vi "FinBuild2.vi"   [LabVIEW 2015]
uses:
  <vilib>/NXT/Block Support/NXT_InputPort.ctl
  <vilib>/NXT/Block Support/NXT_OutputPort.ctl
  <vilib>/NXT/Dual Mode Library/Sensors/Light_On.vi
  <vilib>/NXT/Dual Mode Library/Sensors/Sonar_cm.vi
  <vilib>/NXT/NXTIO Xnodes/NXTIONodeSubVIs/NXTMoveMotors.vi
  <vilib>/NXT/Dual Mode Library/Waits/Wait_Num(msec).vi
  <vilib>/NXT/Subs/LVHSConnector.ctl
  <vilib>/NXT/NXTIO Xnodes/AddressXNode/NXTIOAddress.xnode
  <vilib>/NXT/NXTIO Xnodes/NXTIOXNode/NXTIO.xnode
  <vilib>/NXT/LegoClasses/BrickReference/BrickReference.lvclass
types:
  T1 = typedef "NXT_OutputPort.ctl" = u8
  T2 = typedef "NXT_InputPort.ctl" = u32
  T3 = typedef "LVHSConnector.ctl" = refnum<class "BrickReference.lvclass">
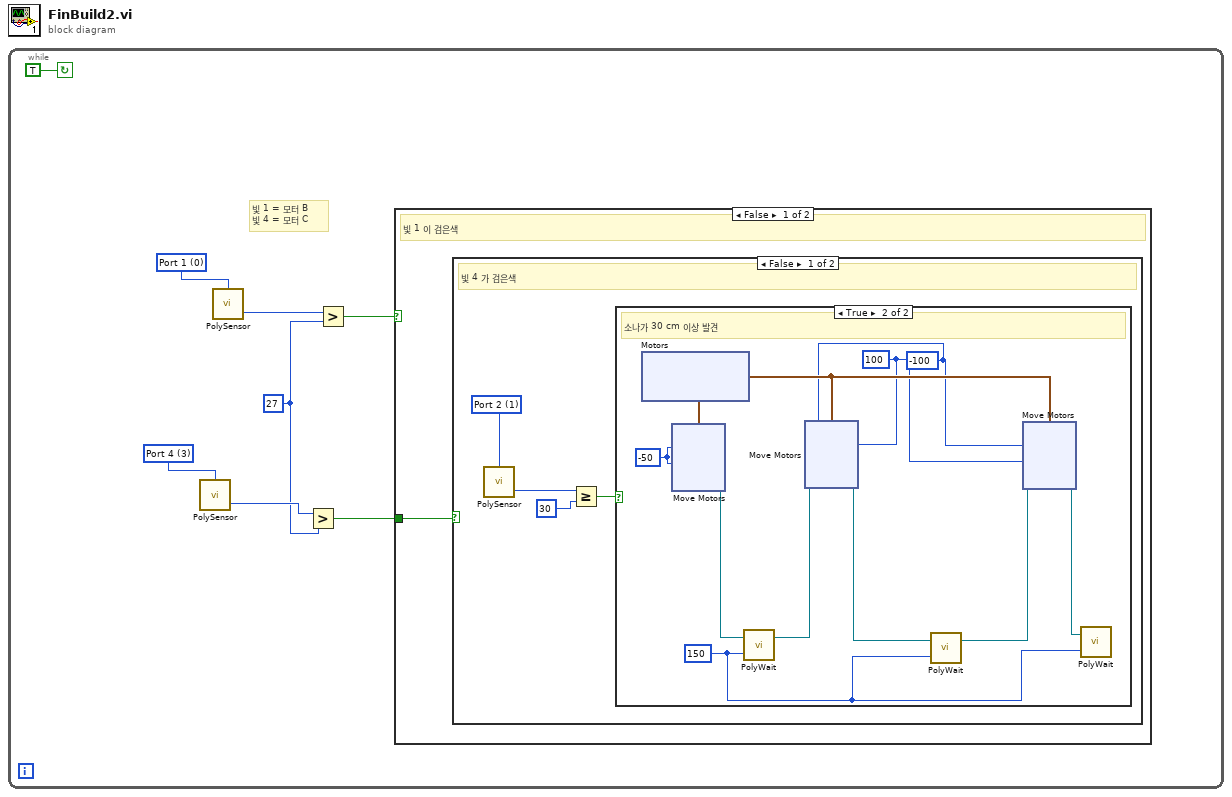
[diagram p0: block diagram]
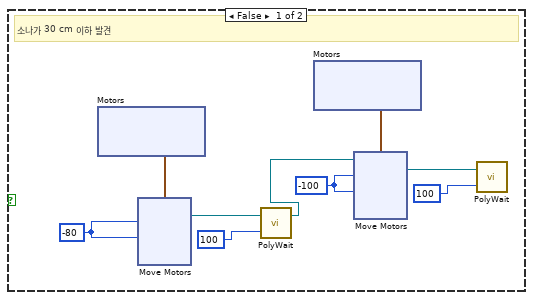
[diagram p2: hidden frame]
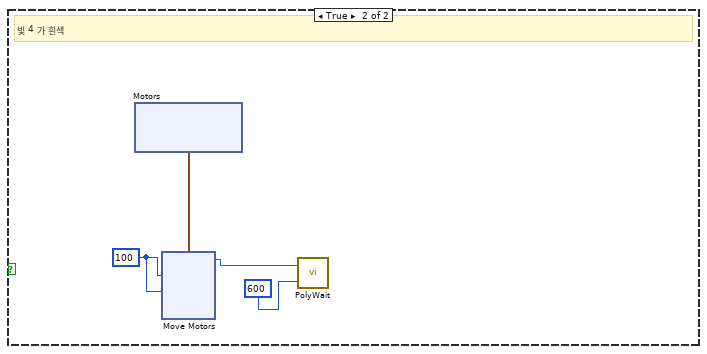
[diagram p3: hidden frame]
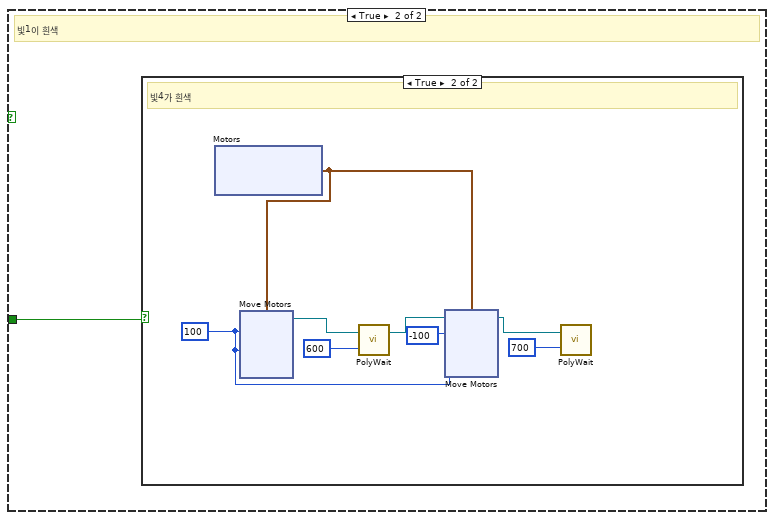
[diagram p4: hidden frame]
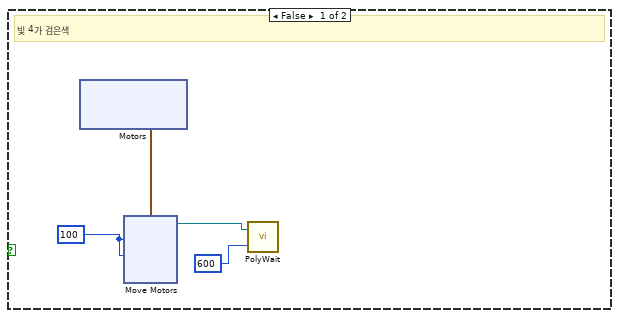
[diagram p5: hidden frame]
diagram:
  n1 = while {
    stop <- TRUE continue-if-true
    w1 = i16 27 ("y")
    w6 = T2 0 items=["Port 1", "Port 2", "Port 3", "Port 4"] ("Port (Port 3)")
    w5 = T2 3 items=["Port 1", "Port 2", "Port 3", "Port 4"] ("Port (Port 3)")
    # "빛 1 = 모터 B\n빛 4 = 모터 C"
    n2 = call-poly <vilib>:"PolySensor.vi"("Port (Port 3)"=w5) -> ("Scaled Value"=w7:i16)  [unwired: 2 in, 1 out]
    n3 = call-poly <vilib>:"PolySensor.vi"("Port (Port 3)"=w6) -> ("Scaled Value"=w8:i16)  [unwired: 2 in, 1 out]
    n4 = Greater?(x=w7, y=w1) -> (0:w3:bool)
    n5 = Greater?(x=w8, y=w1) -> (0:w4:bool)
    n6 = case shown="False" w4 {
      tunnel: w3 -> [w9 w89]
      frame False {
        # "빛 1 이 검은색"
        n7 = case shown="False" w9 {
          frame False {
            w10 = T2 1 items=["Port 1", "Port 2", "Port 3", "Port 4"] ("Port (Port 4)")
            # "빛 4 가 검은색"
            n8 = call-poly <vilib>:"PolySensor.vi"("Port (Port 4)"=w10) -> ("Distance (cm)"=w13:i16)  [unwired: 2 in, 1 out]
            n9 = Greater Or Equal?(x=w13, y=i16 30) -> (x >= y?=w11:bool)
            n10 = case shown="True" w11 {
              frame False {
                w17 = i16 -100 ("y")
                w21 = i16 -80 ("y")
                # "소나가 30 cm 이하 발견"
                n11 = xnode "Motors"() -> ("Motor"=w22:cluster{"Port":T1, "Port":T1})
                n12 = xnode "Move Motors"("Power/Speed 2"=w21, "Power/Speed 1"=w21, "Motors"=w22) -> ("NXT/EV3"=w19:T3)  [unwired: 1 in]
                n13 = call-poly <vilib>:"PolyWait.vi"("Time (100 msec)"=i16 100 ("y"), "NXT/EV3"=w19) -> ("NXT/EV3"=w14:T3)  [unwired: 2 in]
                n14 = xnode "Motors"() -> ("Motor"=w18:cluster{"Port":T1, "Port":T1})
                n15 = xnode "Move Motors"("Power/Speed 2"=w17, "Power/Speed 1"=w17, "Motors"=w18, "NXT/EV3"=w14) -> ("NXT/EV3"=w15:T3)
                n16 = call-poly <vilib>:"PolyWait.vi"("Time (100 msec)"=i16 100 ("y"), "NXT/EV3"=w15) -> ()  [unwired: 2 in, 1 out]
              }
              frame True {
                w42 = i16 -100 ("y")
                w43 = i16 100 ("y")
                w41 = i16 150 ("y")
                w44 = i16 -50 ("y")
                # "소나가 30 cm 이상 발견"
                n17 = xnode "Motors"() -> ("Motor"=w45:cluster{"Port":T1, "Port":T1})
                n18 = xnode "Move Motors"("Power/Speed 2"=w44, "Power/Speed 1"=w44, "Motors"=w45) -> ("NXT/EV3"=w50:T3)  [unwired: 1 in]
                n19 = call-poly <vilib>:"PolyWait.vi"("Time (100 msec)"=w41, "NXT/EV3"=w50) -> ("NXT/EV3"=w49:T3)  [unwired: 2 in]
                n20 = xnode "Move Motors"("Power/Speed 2"=w42, "Power/Speed 1"=w43, "Motors"=w45, "NXT/EV3"=w49) -> ("NXT/EV3"=w48:T3)
                n21 = call-poly <vilib>:"PolyWait.vi"("Time (100 msec)"=w41, "NXT/EV3"=w48) -> ("NXT/EV3"=w47:T3)  [unwired: 2 in]
                n22 = xnode "Move Motors"("Power/Speed 2"=w43, "Power/Speed 1"=w42, "Motors"=w45, "NXT/EV3"=w47) -> ("NXT/EV3"=w46:T3)
                n23 = call-poly <vilib>:"PolyWait.vi"("Time (100 msec)"=w41, "NXT/EV3"=w46) -> ()  [unwired: 2 in, 1 out]
              }
            }
          }
          frame True {
            w76 = i16 100 ("y")
            # "빛 4 가 흰색"
            n24 = xnode "Motors"() -> ("Motor"=w79:cluster{"Port":T1, "Port":T1})
            n25 = xnode "Move Motors"("Power/Speed 2"=w76, "Power/Speed 1"=w76, "Motors"=w79) -> ("NXT/EV3"=w77:T3)  [unwired: 1 in]
            n26 = call-poly <vilib>:"PolyWait.vi"("Time (100 msec)"=i16 600 ("y"), "NXT/EV3"=w77) -> ()  [unwired: 2 in, 1 out]
          }
        }
      }
      frame True {
        # "빛1이 흰색"
        n27 = case shown="True" w89 {
          frame False {
            w90 = i16 100 ("y")
            # "빛 4가 검은색"
            n28 = xnode "Motors"() -> ("Motor"=w93:cluster{"Port":T1, "Port":T1})
            n29 = xnode "Move Motors"("Power/Speed 2"=w90, "Power/Speed 1"=w90, "Motors"=w93) -> ("NXT/EV3"=w91:T3)  [unwired: 1 in]
            n30 = call-poly <vilib>:"PolyWait.vi"("Time (100 msec)"=i16 600 ("y"), "NXT/EV3"=w91) -> ()  [unwired: 2 in, 1 out]
          }
          frame True {
            w103 = i16 100 ("y")
            # "빛4가 흰색"
            n31 = xnode "Motors"() -> ("Motor"=w110:cluster{"Port":T1, "Port":T1})
            n32 = xnode "Move Motors"("Power/Speed 2"=w103, "Power/Speed 1"=w103, "Motors"=w110) -> ("NXT/EV3"=w109:T3)  [unwired: 1 in]
            n33 = call-poly <vilib>:"PolyWait.vi"("Time (100 msec)"=i16 600 ("y"), "NXT/EV3"=w109) -> ("NXT/EV3"=w108:T3)  [unwired: 2 in]
            n34 = xnode "Move Motors"("Power/Speed 2"=w103, "Power/Speed 1"=i16 -100 ("y"), "Motors"=w110, "NXT/EV3"=w108) -> ("NXT/EV3"=w107:T3)
            n35 = call-poly <vilib>:"PolyWait.vi"("Time (100 msec)"=i16 700 ("y"), "NXT/EV3"=w107) -> ()  [unwired: 2 in, 1 out]
          }
        }
      }
    }
  }
